vi "SingleFrame.vi"() -> ()   [LabVIEW 2013]
uses:
  src/Libraries-alpD41/alpD41.lvlib
panel:
  in  "stop 2":bool
  in  "Path to Image":path
  out "Error":T1={"Device Allocation"="ALP_OK", "Height Estimation"="ALP_OK", "Width Estimation"="ALP_OK", "DMD Type Estimation"="ALP_OK", "ALP Seq. Alloc."="ALP_OK", "ALP Bin Mode Alloc."="ALP_OK", "ALP Data Type Alloc."="ALP_OK", "ALP Seq. Repeat"="ALP_OK", "ALP Seq. Timimg"="ALP_OK", "ALP Seq Put"="ALP_OK", "ALP Proj Start"="ALP_OK", "ALP Proj Halt"="ALP_OK", "ALP Seq Free"="ALP_OK", "ALP Dev Free"="ALP_OK"}
  out "Frame Display Properties":T2={"Min. Illuminate Time (us)"=0.0, "Min. Picture Time (us)"=1000000.0}
  out "Error Codes":T3
  out "DMD Characteristics":T4={"Device ID"=343.0, "Height"=768.0, "Width"=1024.0, "DMD Type Code"=4.0, "Sequence ID"=1.0, "DMD Type"="XGA"}
  in  "Advanced Image Display Settings":T5={"PictureTime (ms)"=1000.0, "Time Between Frames  (ms)"=1000.0} {"Time Between Frames  (ms)" min=0.1 max=100.0 step=0.05; "PictureTime (ms)" min=0.3 max=100.0 step=0.1}
  out "error out":errorcluster
  in  "error in (no error)":errorcluster
  # "Basic Inputs"
  # "Debugging"
  # "(Use the STOP button ONLY, not the red dot at the top)"
  # "Display Properties"
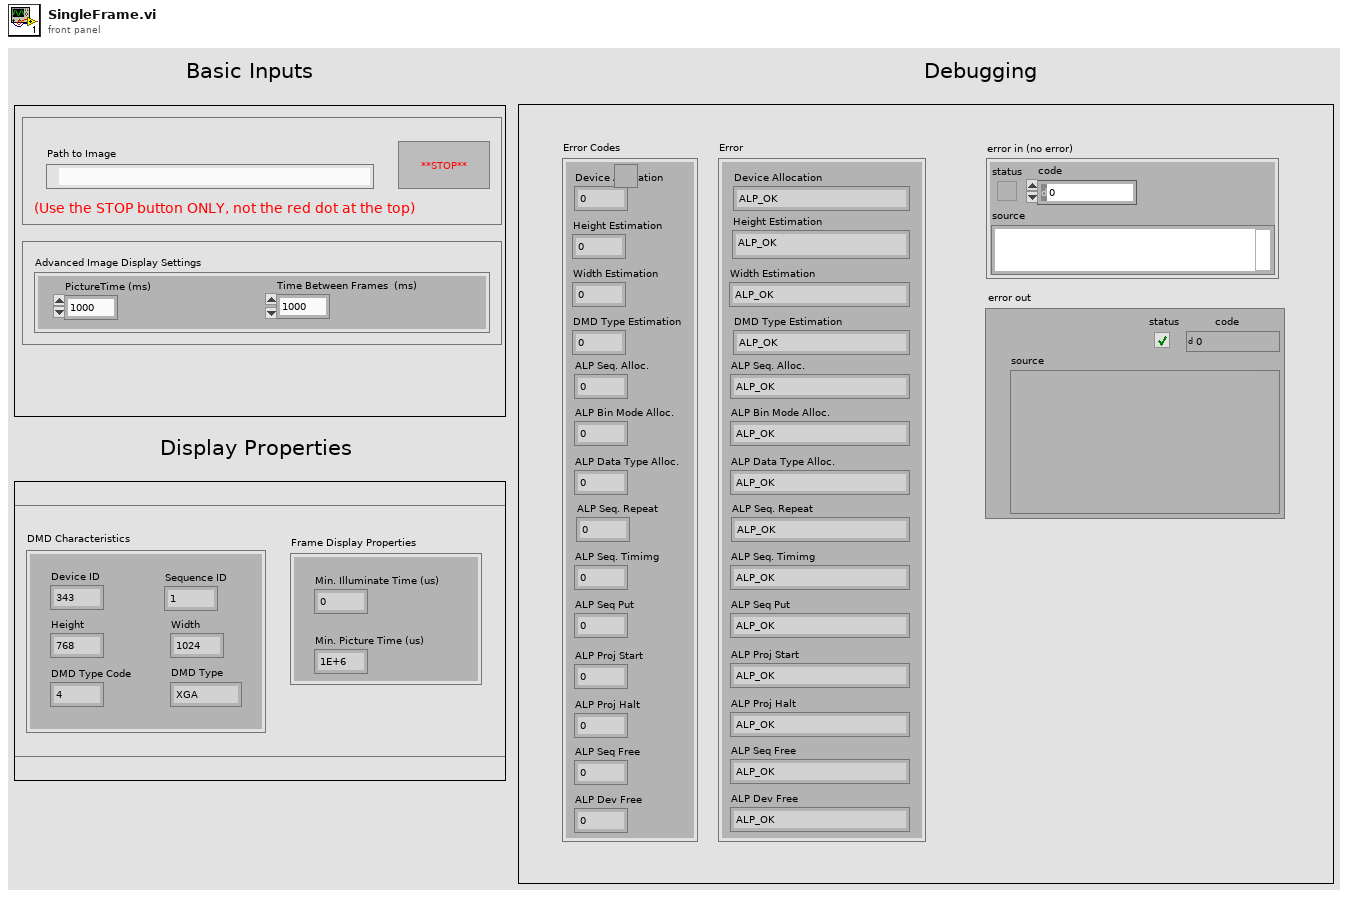
[diagram p1: front panel]
types:
  T1 = cluster{"Device Allocation":string, "Height Estimation":string, "Width Estimation":string, "DMD Type Estimation":string, "ALP Seq. Alloc.":string, "ALP Bin Mode Alloc.":string, "ALP Data Type Alloc.":string, "ALP Seq. Repeat":string, "ALP Seq. Timimg":string, "ALP Seq Put":string, "ALP Proj Start":string, "ALP Proj Halt":string, "ALP Seq Free":string, "ALP Dev Free":string}
  T2 = cluster{"Min. Illuminate Time (us)":dbl, "Min. Picture Time (us)":dbl}
  T3 = cluster{"Device Allocation":dbl, "Height Estimation":dbl, "Width Estimation":dbl, "DMD Type Estimation":dbl, "ALP Seq. Alloc.":dbl, "ALP Bin Mode Alloc.":dbl, "ALP Data Type Alloc.":dbl, "ALP Seq. Repeat":dbl, "ALP Seq. Timimg":dbl, "ALP Seq Put":dbl, "ALP Proj Start":dbl, "ALP Proj Halt":dbl, "ALP Seq Free":dbl, "ALP Dev Free":dbl}
  T4 = cluster{"Device ID":dbl, "Height":dbl, "Width":dbl, "DMD Type Code":dbl, "Sequence ID":dbl, "DMD Type":string}
  T5 = cluster{"PictureTime (ms)":dbl, "Time Between Frames  (ms)":dbl}
  T6 = typedef "imagedata.ctl" = cluster{"image type":i32, "image depth":i32, "image":u8[], "mask":u8[], "colors":u32[], "Rectangle":cluster{"left":i16, "top":i16, "right":i16, "bottom":i16}}
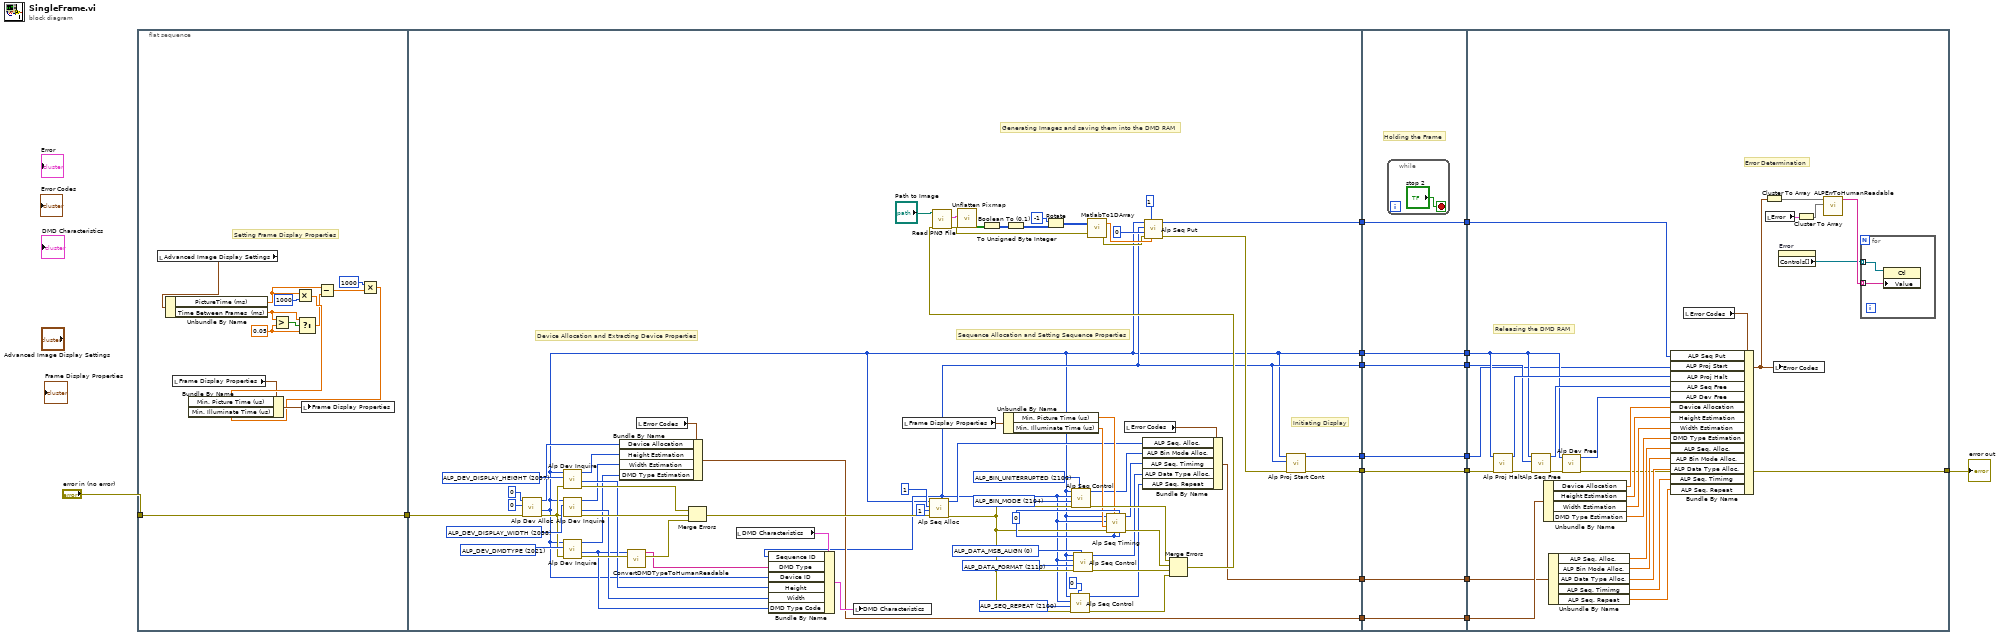
[diagram p0: block diagram]
diagram:
  n1 = flat-sequence {
    tunnel: "error in (no error)" -> [w31]
    tunnel: [w31] -> w16
    tunnel: w16 -> [w88]
    tunnel: [w35] -> w14
    tunnel: [w39] -> w12
    tunnel: [w38] -> w9
    tunnel: [w33] -> w7
    tunnel: [w34] -> w5
    tunnel: [w37] -> w3
    tunnel: [w32] -> w1
    tunnel: w14 -> [w104]
    tunnel: [w104] -> w13
    tunnel: w12 -> [w103]
    tunnel: [w103] -> w11
    tunnel: [w102] -> w10
    tunnel: w9 -> [w102]
    tunnel: [w101] -> w8
    tunnel: w7 -> [w101]
    tunnel: [w100] -> w6
    tunnel: w5 -> [w100]
    tunnel: [w99] -> w4
    tunnel: w3 -> [w99]
    tunnel: [w98] -> w2
    tunnel: w1 -> [w98]
    tunnel: [w108] -> w15
    tunnel: w13 -> [w114]
    tunnel: w11 -> [w113]
    tunnel: w10 -> [w112]
    tunnel: w8 -> [w111]
    tunnel: w6 -> [w110]
    tunnel: w4 -> [w109]
    tunnel: w2 -> [w106]
    frame #0 {
      w25 = 0.05
      # "Setting Frame Display Properties"
      n2 = local read "Advanced Image Display Settings"() -> (w29:T5)
      n3 = Unbundle By Name(w29) -> ("PictureTime (ms)"=w24:dbl, "Time Between Frames  (ms)"=w23:dbl)
      n4 = local read "Frame Display Properties"() -> (w26:T2)
      n5 = Greater?(x=w23, y=w25) -> (0:w19:bool)
      n6 = Multiply(x=w24, y=1000 ("element")) -> (x*y=w28:dbl)
      n7 = Select(t=w23, s=w19, f=w25) -> (s? t:f=w20:dbl)
      n8 = Subtract(x=w24, y=w20) -> (x-y=w21:dbl)
      n9 = Multiply(x=1000, y=w21) -> (x*y=w27:dbl)
      n10 = Bundle By Name(cluster=w26, "Min. Picture Time (us)"=w28, "Min. Illuminate Time (us)"=w27) -> (w30:T2)
      n11 = local write "Frame Display Properties"(w30) -> ()
    }
    frame #1 {
      w67 = u16 2100 items=["ALP_SEQ_REPEAT "=2100, "ALP_FIRSTFRAME"=2101, "ALP_LASTFRAME"=2102, "ALP_BITNUM"=2103, "ALP_BIN_MODE"=2104, "ALP_DATA_FORMAT"=2110, "ALP_SEQ_PUT_LOCK"=2119, "ALP_SCROLL_FROM_ROW"=2123, "ALP_SCROLL_TO_ROW"=2124, "ALP_FIRSTLINE"=2111, "ALP_LASTLINE"=2112, "ALP_LINE_INC"=2113, "ALP_FLUT_MODE"=2118, "ALP_FLUT_EMTRIES9"=2120, "ALP_FLUT_OFFSET9"=2122, "ALP_PWM_MODE"=2107] ("ALPSeqControlType")
      w68 = u16 0 items=["ALP_BIN_NORMAL"=2105, "ALP_BIN_UNITERRUPTED"=2106, "ALP_DATA_MSB_ALIGN"=0, "ALP_DATA_LSB_ALIGN"=1, "ALP_DATA_BINARY_TOPDOWN"=2, "ALP_DATA_BINARY_BOTTOMUP"=3] ("ALPSeqControlValue")
      w69 = u16 2110 items=["ALP_SEQ_REPEAT "=2100, "ALP_FIRSTFRAME"=2101, "ALP_LASTFRAME"=2102, "ALP_BITNUM"=2103, "ALP_BIN_MODE"=2104, "ALP_DATA_FORMAT"=2110, "ALP_SEQ_PUT_LOCK"=2119, "ALP_SCROLL_FROM_ROW"=2123, "ALP_SCROLL_TO_ROW"=2124, "ALP_FIRSTLINE"=2111, "ALP_LASTLINE"=2112, "ALP_LINE_INC"=2113, "ALP_FLUT_MODE"=2118, "ALP_FLUT_EMTRIES9"=2120, "ALP_FLUT_OFFSET9"=2122, "ALP_PWM_MODE"=2107] ("ALPSeqControlType")
      w73 = 0
      w74 = u16 2104 items=["ALP_SEQ_REPEAT "=2100, "ALP_FIRSTFRAME"=2101, "ALP_LASTFRAME"=2102, "ALP_BITNUM"=2103, "ALP_BIN_MODE"=2104, "ALP_DATA_FORMAT"=2110, "ALP_SEQ_PUT_LOCK"=2119, "ALP_SCROLL_FROM_ROW"=2123, "ALP_SCROLL_TO_ROW"=2124, "ALP_FIRSTLINE"=2111, "ALP_LASTLINE"=2112, "ALP_LINE_INC"=2113, "ALP_FLUT_MODE"=2118, "ALP_FLUT_EMTRIES9"=2120, "ALP_FLUT_OFFSET9"=2122, "ALP_PWM_MODE"=2107] ("ControlType")
      w75 = u16 2106 items=["ALP_BIN_NORMAL"=2105, "ALP_BIN_UNITERRUPTED"=2106, "ALP_DATA_MSB_ALIGN"=0, "ALP_DATA_LSB_ALIGN"=1, "ALP_DATA_BINARY_TOPDOWN"=2, "ALP_DATA_BINARY_BOTTOMUP"=3] ("ControlValue")
      w93 = u16 2058 items=["ALP_DEVICE_NUMBER"=2000, "ALP_VERSION"=2001, "ALP_AVAIL_MEMORY"=2003, "ALP_SYNCH_POLARITY"=2004, "ALP_TRIGGER_EDGE"=2005, "ALP_DEV_DMDTYPE"=2021, "ALP_DEV_DISPLAY_HEIGHT"=2057, "ALP_DEV_DISPLAY_WIDTH"=2058, "ALP_USB_CONNECTION"=2016, "ALP_DDC_FPGA_TEMPERATURE"=2050, "ALP_APPS_FPGA_TEMPERATURE"=2051, "ALP_PCB_TEMPERATURE"=2052, "ALP_PWM_LEVEL"=2063] ("InquireType")
      w94 = u16 2057 items=["ALP_DEVICE_NUMBER"=2000, "ALP_VERSION"=2001, "ALP_AVAIL_MEMORY"=2003, "ALP_SYNCH_POLARITY"=2004, "ALP_TRIGGER_EDGE"=2005, "ALP_DEV_DMDTYPE"=2021, "ALP_DEV_DISPLAY_HEIGHT"=2057, "ALP_DEV_DISPLAY_WIDTH"=2058, "ALP_USB_CONNECTION"=2016, "ALP_DDC_FPGA_TEMPERATURE"=2050, "ALP_APPS_FPGA_TEMPERATURE"=2051, "ALP_PCB_TEMPERATURE"=2052, "ALP_PWM_LEVEL"=2063] ("InquireType")
      w97 = u16 2021 items=["ALP_DEVICE_NUMBER"=2000, "ALP_VERSION"=2001, "ALP_AVAIL_MEMORY"=2003, "ALP_SYNCH_POLARITY"=2004, "ALP_TRIGGER_EDGE"=2005, "ALP_DEV_DMDTYPE"=2021, "ALP_DEV_DISPLAY_HEIGHT"=2057, "ALP_DEV_DISPLAY_WIDTH"=2058, "ALP_USB_CONNECTION"=2016, "ALP_DDC_FPGA_TEMPERATURE"=2050, "ALP_APPS_FPGA_TEMPERATURE"=2051, "ALP_PCB_TEMPERATURE"=2052, "ALP_PWM_LEVEL"=2063] ("InquireType")
      # "Initiating Display"
      # "Generating Images and saving them into the DMD RAM"
      # "Sequence Allocation and Setting Sequence Properties"
      # "Device Allocation and Extracting Device Properties"
      n12 = call "Alp Dev Alloc.vi"("error in (no error)"=w88, "InitFlag"=0 ("DeviceNum"), "DeviceNum"=0) -> ("error out"=w92:errorcluster, "DeviceIdPtr out"=w33:u32, "function return"=w81:i32)  [unwired: 6 in]
      n13 = call "Alp Dev Inquire.vi"("error in (no error)"=w92, "InquireType"=w94, "DeviceId"=w33) -> ("error out"=w91:errorcluster, "UserVarPtr out"=w86:i32, "function return"=w80:i32)  [unwired: 6 in]
      n14 = call "Alp Dev Inquire.vi"("error in (no error)"=w92, "InquireType"=w93, "DeviceId"=w33) -> ("error out"=w90:errorcluster, "UserVarPtr out"=w85:i32, "function return"=w79:i32)  [unwired: 6 in]
      n15 = call "Alp Dev Inquire.vi"("error in (no error)"=w92, "InquireType"=w97, "DeviceId"=w33) -> ("error out"=w89:errorcluster, "UserVarPtr out"=w84:i32, "function return"=w78:i32)  [unwired: 6 in]
      n16 = call "ConvertDMDTypeToHumanReadable.vi"("UserVarPtr in"=w84) -> ("String"=w83:string)  [unwired: 10 in]
      n17 = local read "Error Codes"() -> (w82:T3)
      n18 = Bundle By Name(cluster=w82, "Device Allocation"=w81, "Height Estimation"=w80, "Width Estimation"=w79, "DMD Type Estimation"=w78) -> (w39:T3)
      n19 = Merge Errors(w91, w90, w89) -> (w56:errorcluster)
      n20 = local read "DMD Characteristics"() -> (w87:T4)
      n21 = local read "Frame Display Properties"() -> (w55:T2)
      n22 = call "Alp Seq Alloc.vi"("error in (no error)"=w56, "PicNum"=1, "BitPlanes"=1, "DeviceId"=w33) -> ("error out"=w66:errorcluster, "function return"=w61:i32, "SequenceIdPtr out"=w34:u32)  [unwired: 5 in]
      n23 = Bundle By Name(cluster=w87, "Sequence ID"=w34, "DMD Type"=w83, "Device ID"=w33, "Height"=w86, "Width"=w85, "DMD Type Code"=w84) -> (w77:T4)
      n24 = local write "DMD Characteristics"(w77) -> ()
      n25 = Unbundle By Name(w55) -> ("Min. Picture Time (us)"=w64:dbl, "Min. Illuminate Time (us)"=w63:dbl)
      n26 = call "Alp Seq Control.vi"("ControlValue"=0, "error in (no error)"=w66, "ControlType"=w67, "SequenceId"=w34, "DeviceId"=w33) -> ("error out"=w65:errorcluster, "function return"=w57:i32)  [unwired: 5 in]
      n27 = call "Alp Seq Control.vi"("ControlValue"=w75, "error in (no error)"=w66, "ControlType"=w74, "SequenceId"=w34, "DeviceId"=w33) -> ("error out"=w72:errorcluster, "function return"=w60:i32)  [unwired: 5 in]
      n28 = call "Alp Seq Control.vi"("ControlValue"=w68, "error in (no error)"=w66, "ControlType"=w69, "SequenceId"=w34, "DeviceId"=w33) -> ("error out"=w70:errorcluster, "function return"=w58:i32)  [unwired: 5 in]
      n29 = call "Alp Seq Timing.vi"("TriggerInDelay"=w73, "SynchPulseWidth"=w73, "SynchDelay"=w73, "PictureTime"=w64, "error in (no error)"=w66, "IlluminateTime"=w63, "SequenceId"=w34, "DeviceId"=w33) -> ("error out"=w71:errorcluster, "function return"=w59:i32)  [unwired: 2 in]
      n30 = local read "Error Codes"() -> (w62:T3)
      n31 = Bundle By Name(cluster=w62, "ALP Seq. Alloc."=w61, "ALP Bin Mode Alloc."=w60, "ALP Seq. Timimg"=w59, "ALP Data Type Alloc."=w58, "ALP Seq. Repeat"=w57) -> (w38:T3)
      n32 = Merge Errors(w72, w71, w70, w65) -> (w46:errorcluster)
      n33 = call <vilib>:"Read PNG File.vi"("error in (no error)"=w46, "path to PNG file"="Path to Image") -> ("error out"=w43:errorcluster, "image data"=w51:T6)  [unwired: 7 in, 1 out]
      n34 = call <vilib>:"Unflatten Pixmap.vi"("image data"=w51) -> ("1-bit pixmap"=w49:bool[][])  [unwired: 4 in, 6 out]
      n35 = Boolean To (0,1)(Boolean=w49) -> (0, 1=w50:i16[][])
      n36 = To Unsigned Byte Integer(number=w50) -> (unsigned 8bit integer=w48:u8[][])
      n37 = Rotate(1:w48, 2:-1) -> (0:w45:u8[][])
      n38 = call "MatlabTo1DArray.vi"("error in (no error)"=w43, "Array In"=w45) -> ("error out"=w42:errorcluster, "Array Out"=w44:dbl[])
      n39 = call "Alp Seq Put.vi"("UserArrayPtr"=w44, "PicLoad"=1, "error in (no error)"=w42, "PicOffset"=0, "SequenceId"=w34, "DeviceId"=w33) -> ("error out"=w36:errorcluster, "function return"=w37:i32)  [unwired: 3 in, 1 out]
      n40 = call "Alp Proj Start Cont.vi"("error in (no error)"=w36, "SequenceId"=w34, "DeviceId"=w33) -> ("error out"=w35:errorcluster, "function return"=w32:i32)  [unwired: 7 in]
    }
    frame #2 {
      # "Holding the Frame"
      n41 = while {
        stop <- "stop 2" stop-if-true
      }
    }
    frame #3 {
      # "Error Determination"
      # "Releasing the DMD RAM"
      n42 = call "Alp Proj Halt.vi"("error in (no error)"=w114, "DeviceId"=w111) -> ("error out"=w129:errorcluster, "function return"=w127:i32)  [unwired: 8 in]
      n43 = call "Alp Seq Free.vi"("error in (no error)"=w129, "SequenceId"=w110, "DeviceId"=w111) -> ("error out"=w130:errorcluster, "function return"=w126:i32)  [unwired: 7 in]
      n44 = Unbundle By Name(w113) -> ("Device Allocation"=w123:dbl, "Height Estimation"=w122:dbl, "Width Estimation"=w121:dbl, "DMD Type Estimation"=w120:dbl)
      n45 = Unbundle By Name(w112) -> ("ALP Seq. Alloc."=w119:dbl, "ALP Bin Mode Alloc."=w118:dbl, "ALP Data Type Alloc."=w117:dbl, "ALP Seq. Timimg"=w116:dbl, "ALP Seq. Repeat"=w115:dbl)
      n46 = call "Alp Dev Free.vi"("error in (no error)"=w130, "DeviceId"=w111) -> ("error out"=w108:errorcluster, "function return"=w125:i32)  [unwired: 8 in]
      n47 = local read "Error Codes"() -> (w128:T3)
      n48 = Bundle By Name(cluster=w128, "ALP Seq Put"=w109, "ALP Proj Start"=w106, "ALP Proj Halt"=w127, "ALP Seq Free"=w126, "ALP Dev Free"=w125, "Device Allocation"=w123, "Height Estimation"=w122, "Width Estimation"=w121, "DMD Type Estimation"=w120, "ALP Seq. Alloc."=w119, "ALP Bin Mode Alloc."=w118, "ALP Data Type Alloc."=w117, "ALP Seq. Timimg"=w116, "ALP Seq. Repeat"=w115) -> (w124:T3)
      n49 = Cluster To Array(cluster=w124) -> (array=w132:dbl[])
      n50 = local read "Error"() -> (w134:T1)
      n51 = local write "Error Codes"(w124) -> ()
      n52 = property on="Error" class="Clust (strict)"() -> ("Controls[]"=w107:refnum<vi>[])  [unwired: 2 in, 2 out]
      n53 = Cluster To Array(cluster=w134) -> (array=w133:string[])
      n54 = call "ALPErrToHumanReadable.vi"("Error In"=w133, "Error Codes"=w132) -> ("Error Out"=w131:string[])  [unwired: 9 in]
      n55 = for {
        tunnel: w107 -> [w136] mode=indexing
        tunnel: w131 -> [w135] mode=indexing
        n56 = property class="Ctl"(reference=w136, "Value"=w135) -> ()  [unwired: 1 in, 2 out]
      }
    }
  }
  "error out" <- w15
